vi "LVProjectShortcut_FileSelectionModeGlobal.vi"(7 "Set":enum16{"Set", "Get"}(ring)=enum."Get", 8 "error in":errorcluster, 10 "files in libraries":bool) -> (0 "error out":errorcluster, 2 "files in libraries out":bool, 3 "Selection Mode":T1(ring))   [LabVIEW 2017, in "LVProject Shortcut.lvlib"]
doc: "Gets or Sets the Selection Mode."
uses:
  LVProject Shortcut.lvlib
  <vilib>/UserTags/UserTags.lvlib
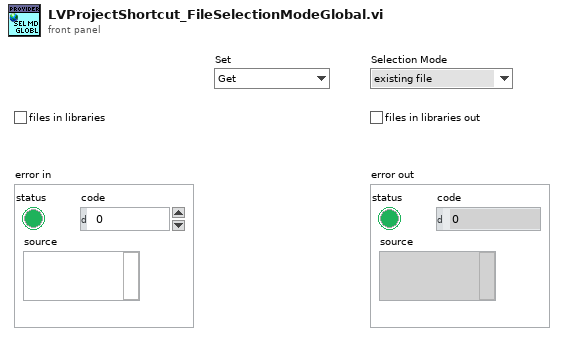
[diagram p1: front panel]
types:
  T1 = enum32{"existing file", "new file", "new or existing file", "existing dir", "new dir", "new or existing dir", "existing file (use LLBs)", "new file (use LLBs)", "new or existing file (use LLBs)", "new or existing file or directory (use LLBs)", "existing dir (use LLBs)", "new dir (use LLBs)", "new or existing dir (use LLBs)", "existing file or dir", "new file or dir", "new or existing file or dir", "existing file or dir (use LLBs)", "new file or dir (use LLBs)"}
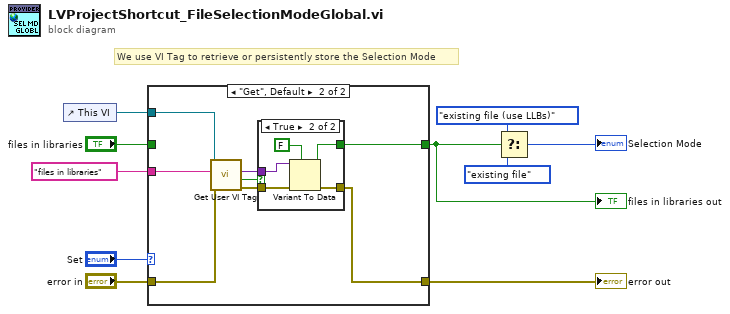
[diagram p0: block diagram]
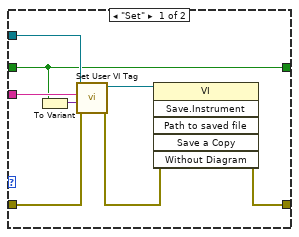
[diagram p2: hidden frame]
diagram:
  # "We use VI Tag to retrieve or persistently store the Selection Mode"
  n1 = control-ref of="This VI"() -> (w6:refnum<vi>)
  n2 = case shown="\"Get\", Default" "Set" {
    tunnel: [w18 w20] -> w10
    tunnel: "files in libraries" -> [w11 _]
    tunnel: "error in" -> [w14 w24]
    tunnel: w6 -> [w13 w26]
    tunnel: "files in libraries" ("Tag Name") -> [w12 w25]
    tunnel: [w11 w19] -> w1
    frame "Set" {
      n3 = To Variant(anything=w11) -> (Variant=w17:variant)
      n4 = call <vilib>:"Set User VI Tag.vi"("error in (no error)"=w14, "Value"=w17, "Tag Name"=w12, "VI Refnum"=w13) -> ("error out"=w15:errorcluster, "dup VI Refnum"=w16:refnum<vi>)  [unwired: 5 in, 1 out]
      n5 = invoke class="VI" method="Save.Instrument"(reference=w16, error in=w15) -> (error out=w18:errorcluster)  [unwired: 4 in, 5 out]
    }
    frame "Get", Default {
      n6 = call <vilib>:"Get User VI Tag.vi"("error in (no error)"=w24, "Tag Name"=w25, "VI Refnum"=w26) -> ("error out"=w21:errorcluster, "Was Tag Found?"=w22:bool, "Value"=w23:variant)  [unwired: 5 in, 1 out]
      n7 = case shown="True" w22 {
        tunnel: w23 -> [_ w32]
        tunnel: w21 -> [w27 w30]
        tunnel: [_ w29] -> w19
        tunnel: [w27 w28] -> w20
        frame False {
        }
        frame True {
          n8 = Variant To Data(error in=w30, type=FALSE, Variant=w32) -> (data=w29:bool, error out=w28:errorcluster)
        }
      }
    }
  }
  "error out" <- w10
  "files in libraries out" <- w1
  n9 = Select(t=T1."existing file (use LLBs)" ("Browse Options:Selection Mode"), s=w1, f=T1."existing file" ("Browse Options:Selection Mode")) -> (s? t:f=→"Selection Mode":T1)
